vi "Calculate Position Orientation 3.vi"(8 "error in":errorcluster, 10 "Fiducials":T1[](array[typedef]), 11 "Feature Definitions":T5(array[cluster])) -> (0 "error out":errorcluster, 3 "PositionOrientation":T6)   [LabVIEW 2023]
uses:
  Vec3d Class/Vec3d.lvclass
  Orient3d Class/Orient3d.lvclass
  Type Definitions/Position_Orientation.ctl
  <vilib>/vision/Image Controls.llb/IMAQ Image.ctl
  Type Definitions/Physical Image.ctl
  Type Definitions/Fiducial with Source.ctl
  Type Definitions/Fiducial Image.ctl
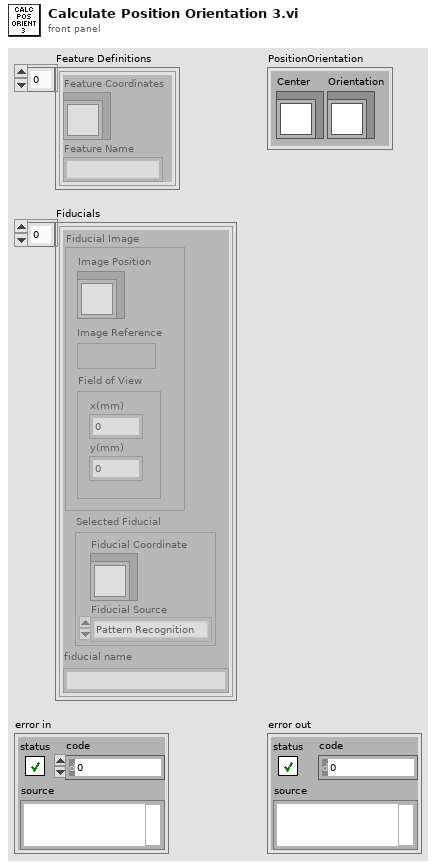
[diagram p1: front panel]
types:
  T1 = typedef "Fiducial Image.ctl" = cluster{"Fiducial Image":T2, "Selected Fiducial":T4, "fiducial name":string}
  T2 = typedef "Physical Image.ctl" = cluster{"Image Position":refnum<class "Vec3d.lvclass">, "Image Reference":T3, "Field of View":cluster{"x(mm)":dbl, "y(mm)":dbl}}
  T3 = typedef "IMAQ Image.ctl" = refnum<image>
  T4 = typedef "Fiducial with Source.ctl" = cluster{"Fiducial Coordinate":refnum<class "Vec3d.lvclass">, "Fiducial Source":enum16{"Pattern Recognition", "User", "Error", "Default"}}
  T5 = cluster{"Feature Coordinates":refnum<class "Vec3d.lvclass">, "Feature Name":string}[]
  T6 = typedef "Position_Orientation.ctl" = cluster{"Center":refnum<class "Vec3d.lvclass">, "Orientation":refnum<class "Orient3d.lvclass">}
  T7 = cluster{"Feature Coordinates":refnum<class "Vec3d.lvclass">, "Feature Name":string}
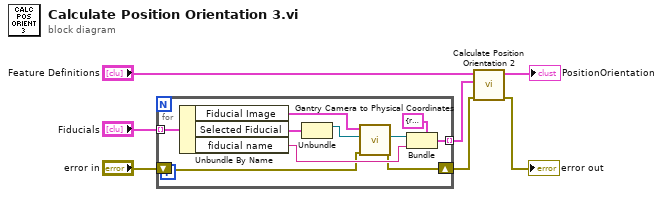
[diagram p0: block diagram]
diagram:
  n1 = for {
    tunnel: "Fiducials" -> [w17] mode=indexing
    tunnel: [w10] -> w3 mode=indexing
    shift-right: [w8] -> w5
    shift-left: "error in" -> [w9]
    n2 = Unbundle By Name(w17) -> ("Fiducial Image"=w15:T2, "Selected Fiducial"=w16:T4, "fiducial name"=w11:string)
    n3 = Unbundle(w16) -> ("Fiducial Coordinate"=w14:refnum<class "Vec3d.lvclass">)  [unwired: 1 out]
    n4 = call "Gantry Camera to Physical Coordinates.vi"("error in"=w9, "Image Coordinate"=w14, "Physical Image"=w15) -> ("error out"=w8:errorcluster, "Global Coordinate"=w12:refnum<class "Vec3d.lvclass">)  [unwired: 6 in, 1 out]
    n5 = Bundle(cluster=T7 {"Feature Coordinates"=refnum, "Feature Name"=""} ("Feature Description"), "Feature Coordinates"=w12, "Feature Name"=w11) -> (w10:T7)
  }
  n6 = call "Calculate Position Orientation 2.vi"("error in"=w5, "Measured Global Positions"=w3, "Known Local Positions"="Feature Definitions") -> ("error out"=→"error out":errorcluster, "PositionOrientation"=→"PositionOrientation":T6)  [unwired: 6 in, 1 out]
